vi "frequency_sweep_2.vi"() -> ()   [LabVIEW 2016]
uses:
  controls/State.ctl
  controls/Data.ctl
  <vilib>/Utility/error.llb/DialogType.ctl
  <vilib>/DAQmx/write.llb/DAQmx Write (Analog DBL 1Chan 1Samp).vi
  <vilib>/DAQmx/create/channels.llb/DAQmx Create Channel (AO-Voltage-Basic).vi
  <vilib>/DAQmx/miscellaneous.llb/DAQmx Fill In Error Info.vi
  <instrlib>/niVNA/niVNA.llb/niVNA Fetch Sweep Measurement (DBL).vi
panel:
  out "DAQ channel Out":tag="DAQ_6363/ao0"
  in  "Averaging Points":i32=4 min=1 max=3201 step=1
  in  "DAQ channel In":tag="DAQ_6363/ao0"
  in  "Exit Button":bool
  in  "IF Bandwidth":dbl(ring)=1000.0 items=["10 Hz"=10.0, "30 Hz"=30.0, "100 Hz"=100.0, "300 Hz"=300.0, "1 KHz"=1000.0, "3 KHz"=3000.0, "10 KHz"=10000.0, "30 KHz"=30000.0]
  in  "Reference H Field (Oe)":dbl=5500.0 min=-6000.0 max=6000.0
  in  "H Field (Oe)":dbl=1000.0 min=-6000.0 max=6000.0
  in  "Save Button":bool
  out "Status":string="Shutting down...Sweeping field to zero..."
  out "Cursor":cluster{"x":dbl, "y":dbl} {"x" format="%.2f"; "y" format="%.5f"}
  out "VNA Name Out":refnum<k15>="VNA_5630"
  out "Error Out":errorcluster
  in  "Error In (no error)":errorcluster
  in  "Format":i32(ring)=1 items=["Log Magnitude (dB)"=0, "Lin Magnitude"=1, "Phase (deg)"=2, "VSWR"=3, "Group Delay"=6]
  out "SpectrumGraph":cluster{"Field":dbl[], "Signal":dbl[]}(graph)
  in  "S-parameter":i32(ring)=1 caption="Measurement" items=["S11", "S21"]
  in  "Start Button":bool
  in  "Stop Button":bool
  in  "Output Power (dBm)":dbl=1.0 min=-25.0 max=5.0 step=0.5
  in  "Number of Points":i32=1000 min=1 max=3201 step=1
  in  "Stop frequency (GHz)":dbl=6.0 caption="Stop H Field (Oe)" min=0.01 max=6.0 format="%#_6f"
  in  "Start frequency (GHz)":dbl=1.0 min=0.01 max=6.0 format="%#_6f"
  in  "VNA Name In":refnum<k15>="VNA_5630"
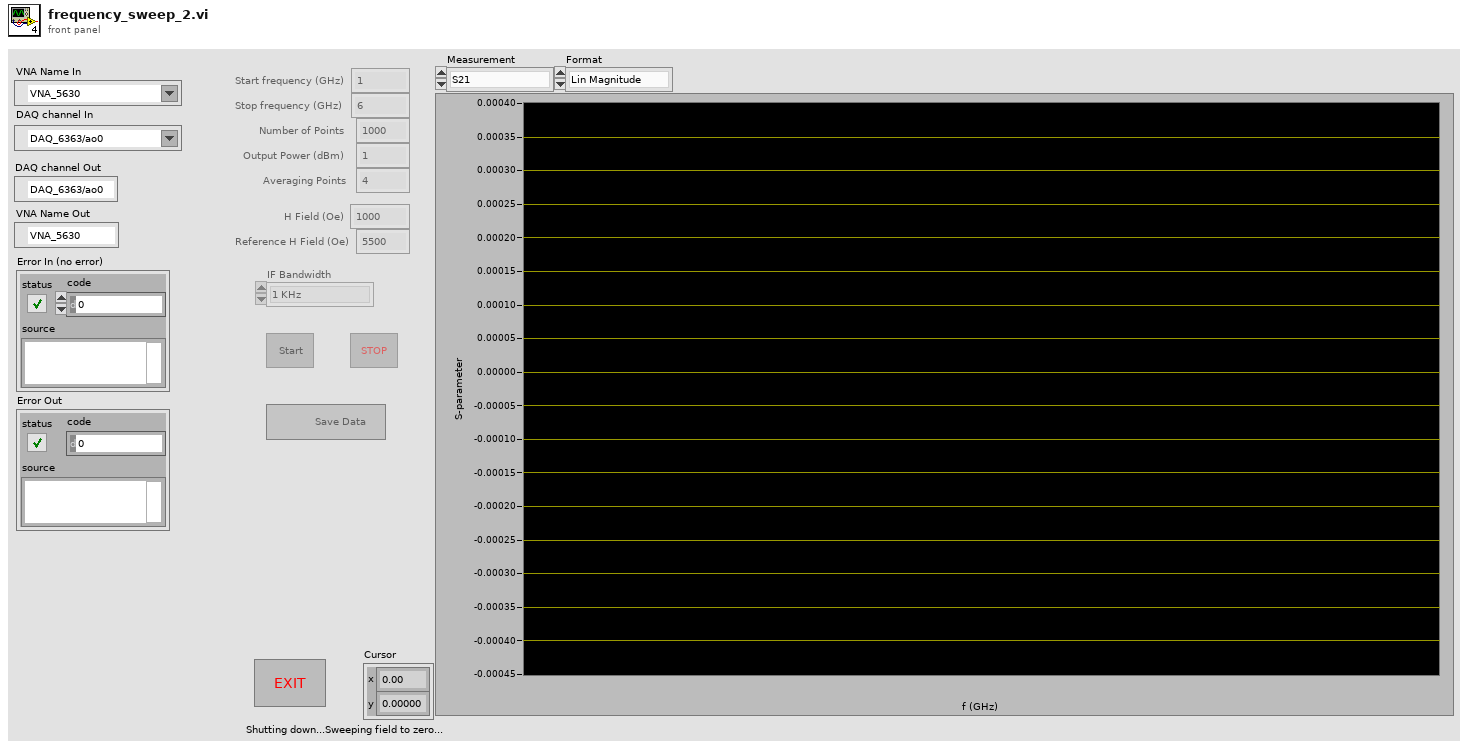
[diagram p1: front panel]
types:
  T1 = typedef "Data.ctl" = cluster{"Frequency":dbl[], "Signal":dbl[], "Ref signal":dbl[]}
  T2 = typedef "State.ctl" = enum16{"Init", "Idle", "Sweeping to ref", "Measuring ref", "Sweeping to H", "Measuring H", "Sweeping down", "Shutdown"}
  T3 = typedef "DialogType.ctl" = u16
  T4 = typedef "LVPoint32TypeDef.ctl" = cluster{"Horizontal":i32, "Vertical":i32}
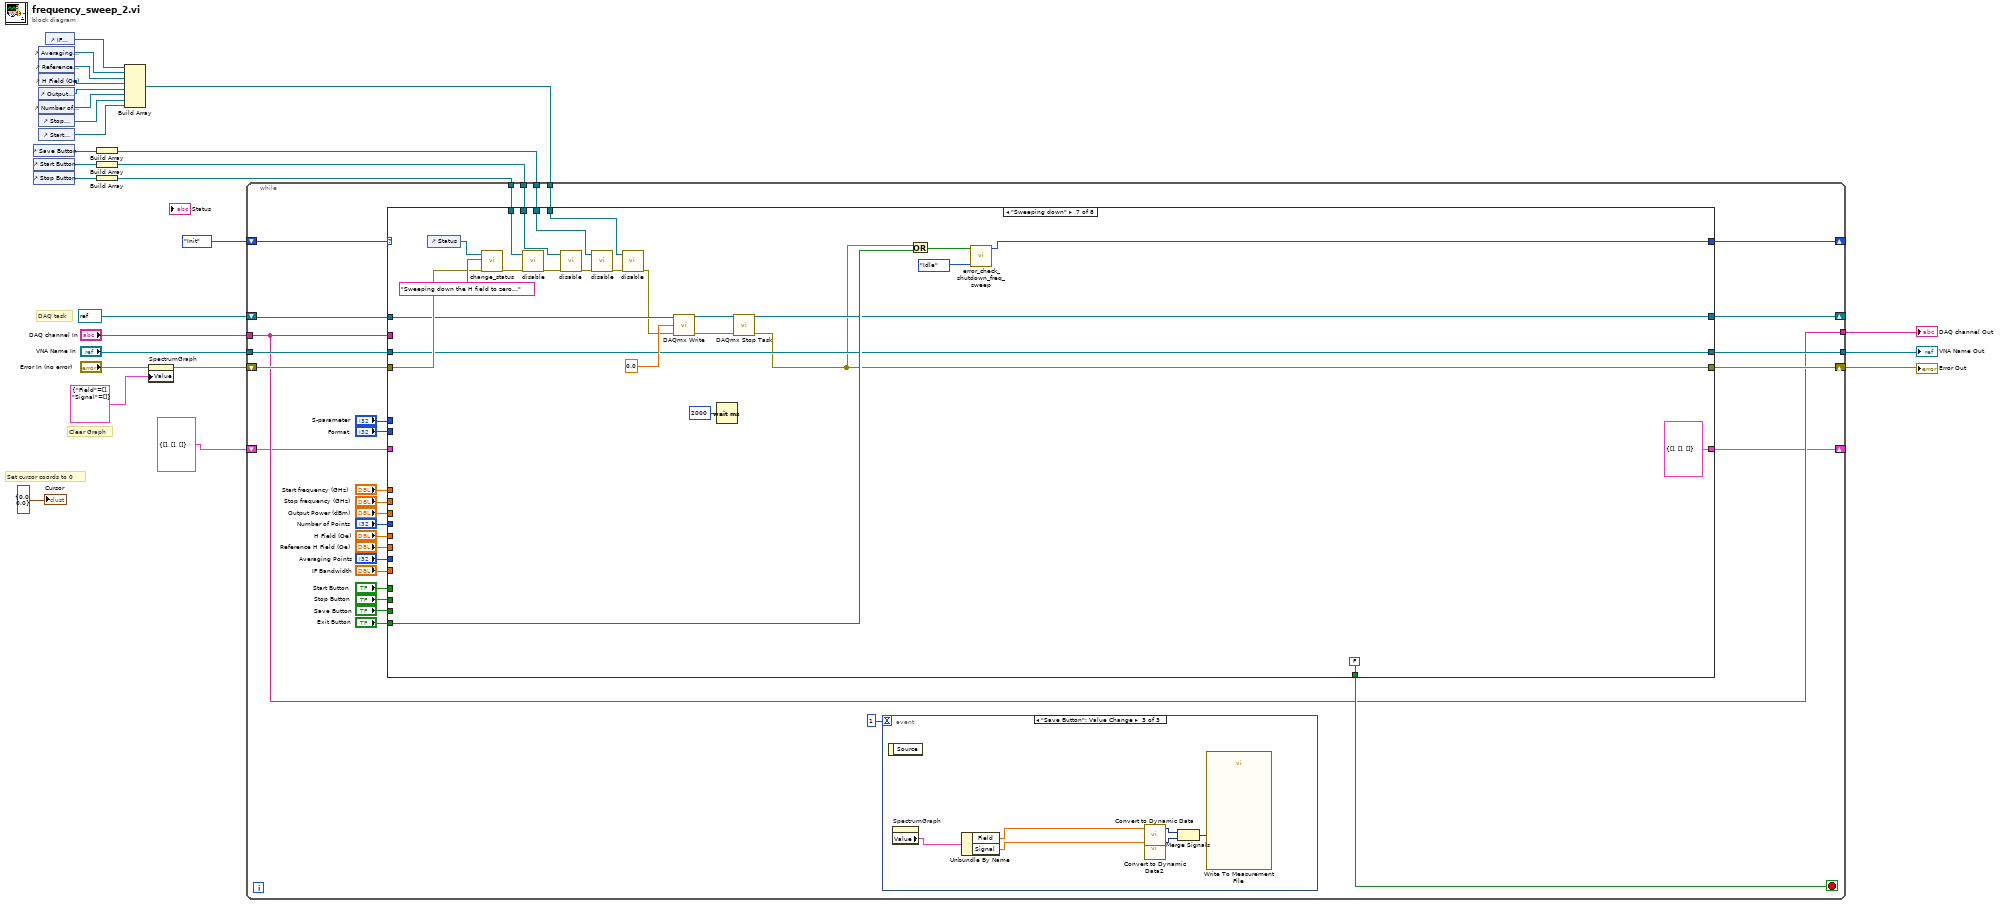
[diagram p0: block diagram]
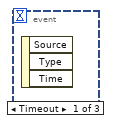
[diagram p2: hidden frame]
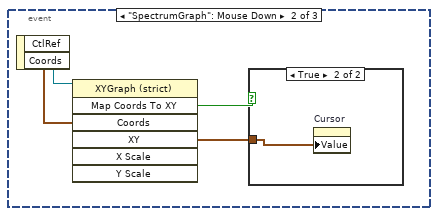
[diagram p3: hidden frame]
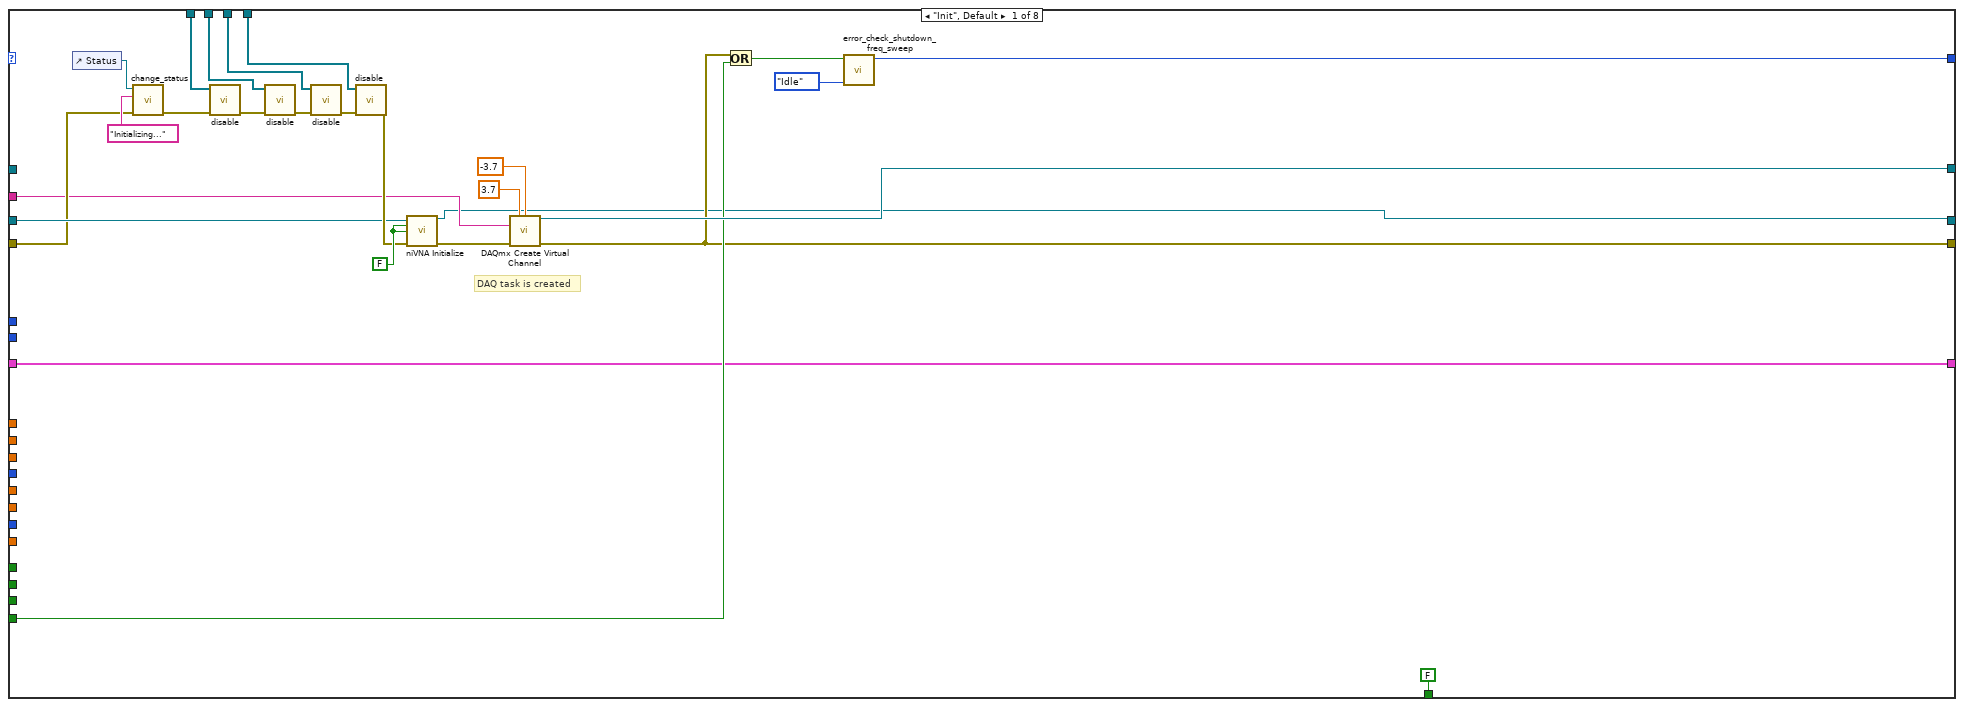
[diagram p5: hidden frame]
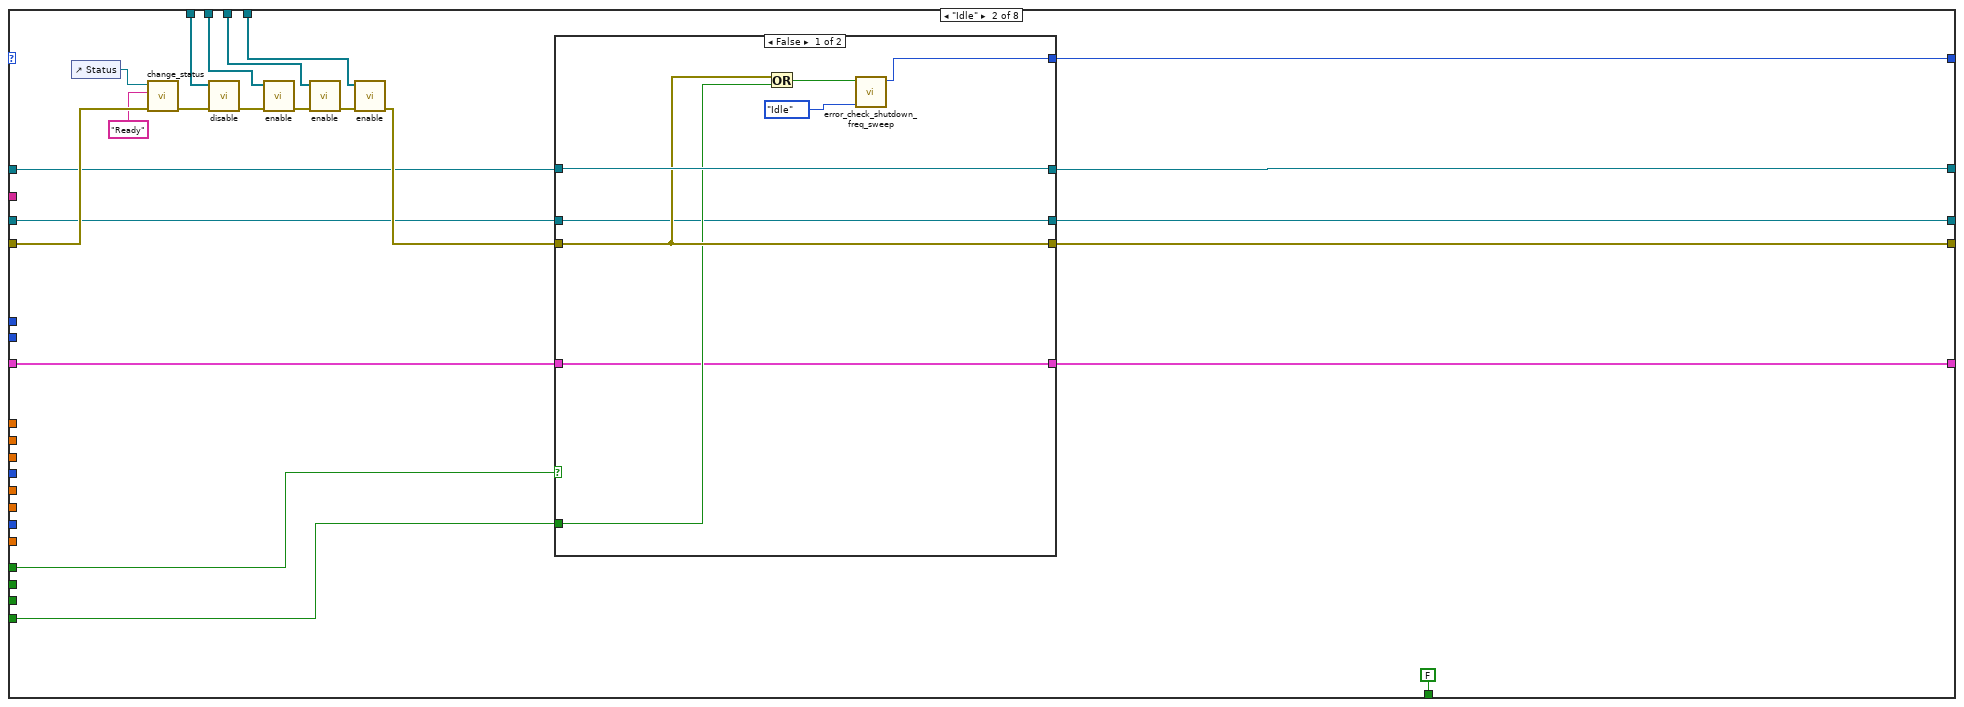
[diagram p6: hidden frame]
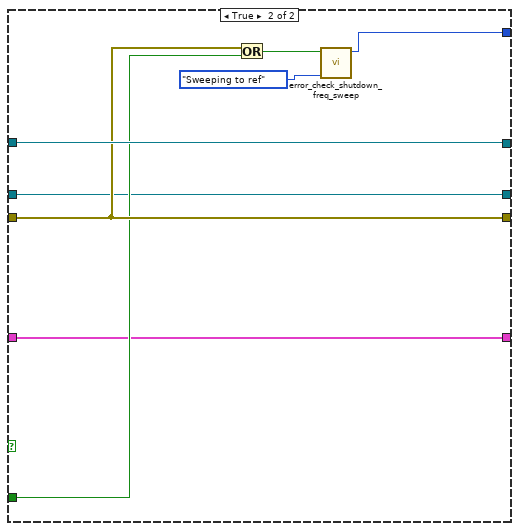
[diagram p7: hidden frame]
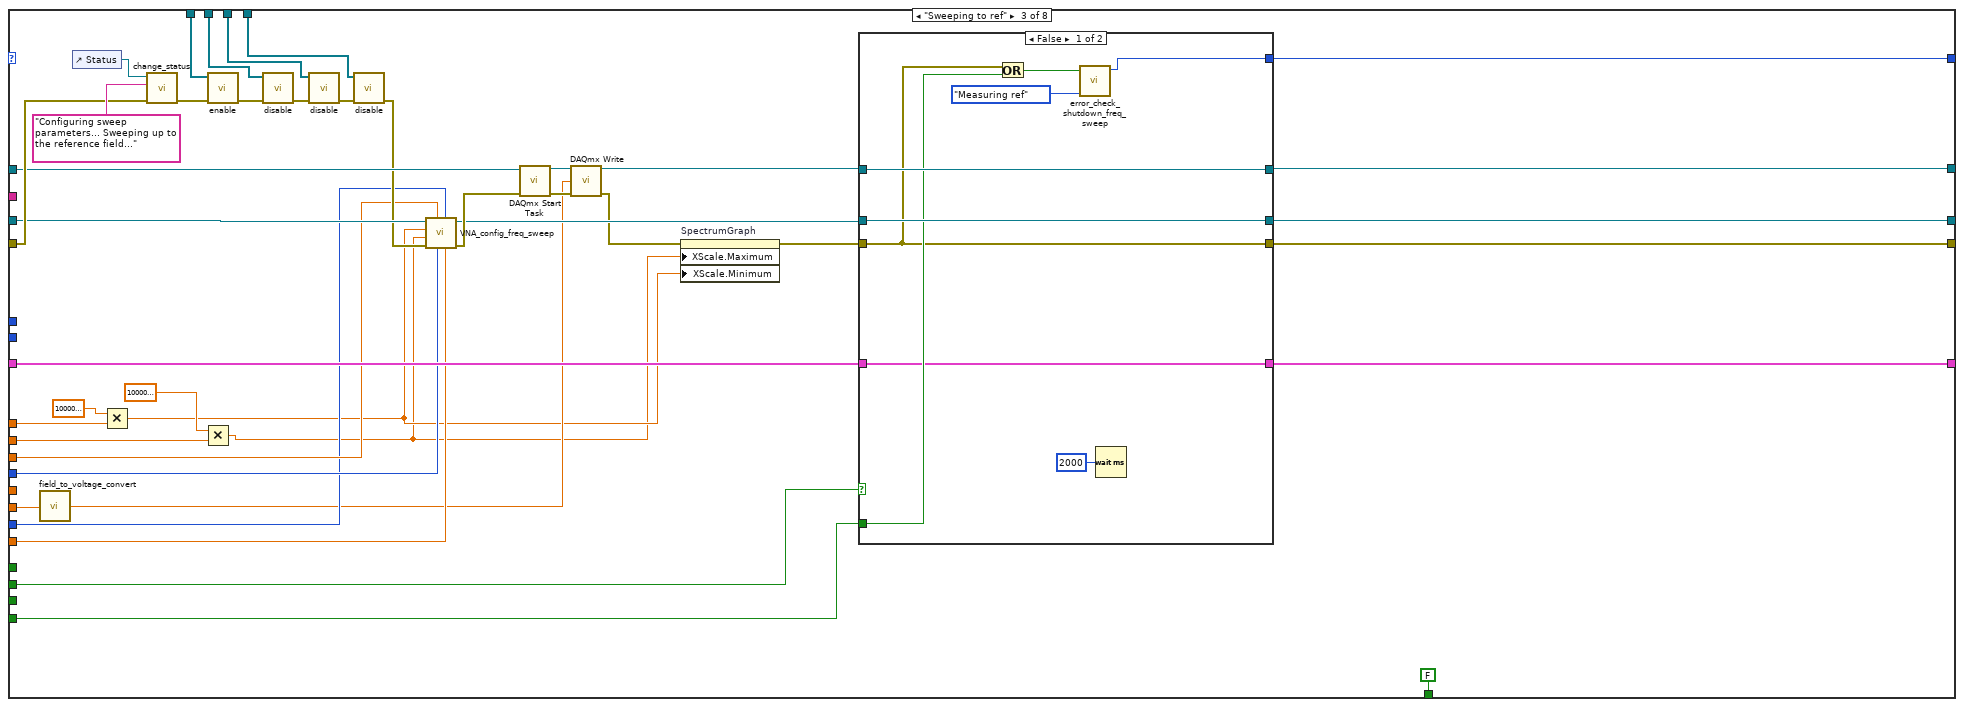
[diagram p8: hidden frame]
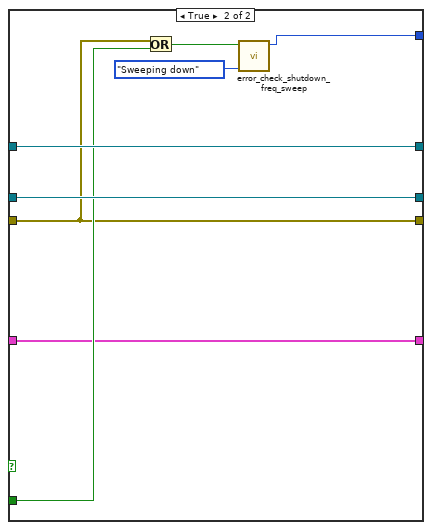
[diagram p9: hidden frame]
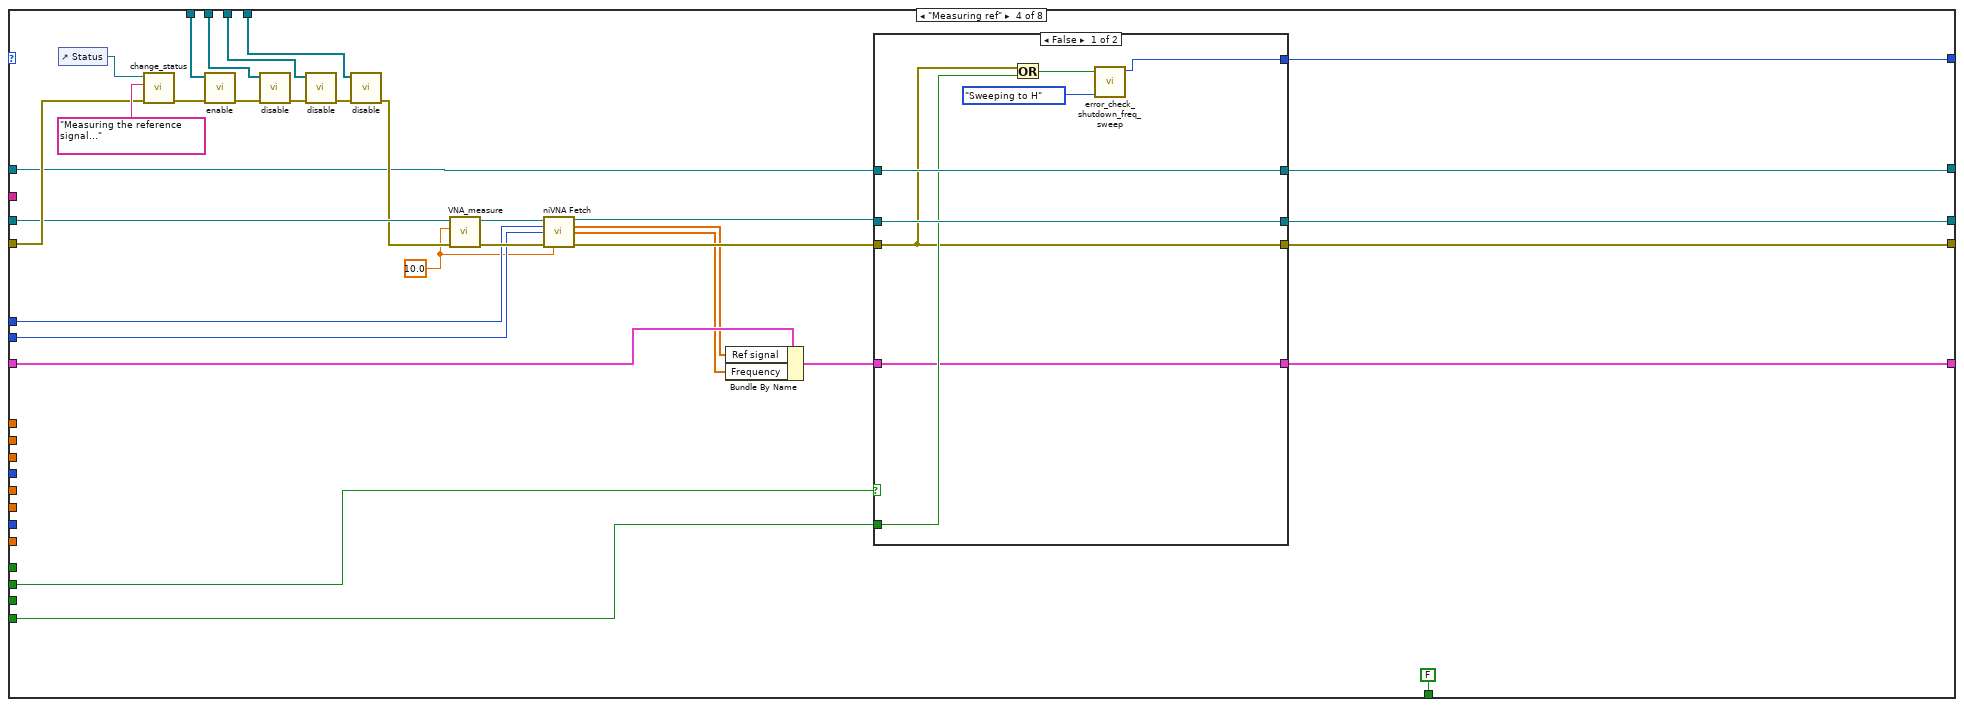
[diagram p10: hidden frame]
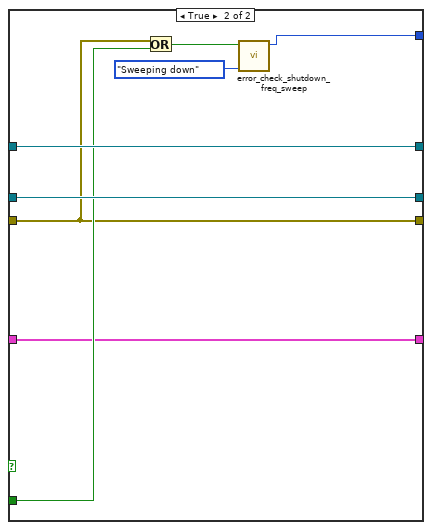
[diagram p11: hidden frame]
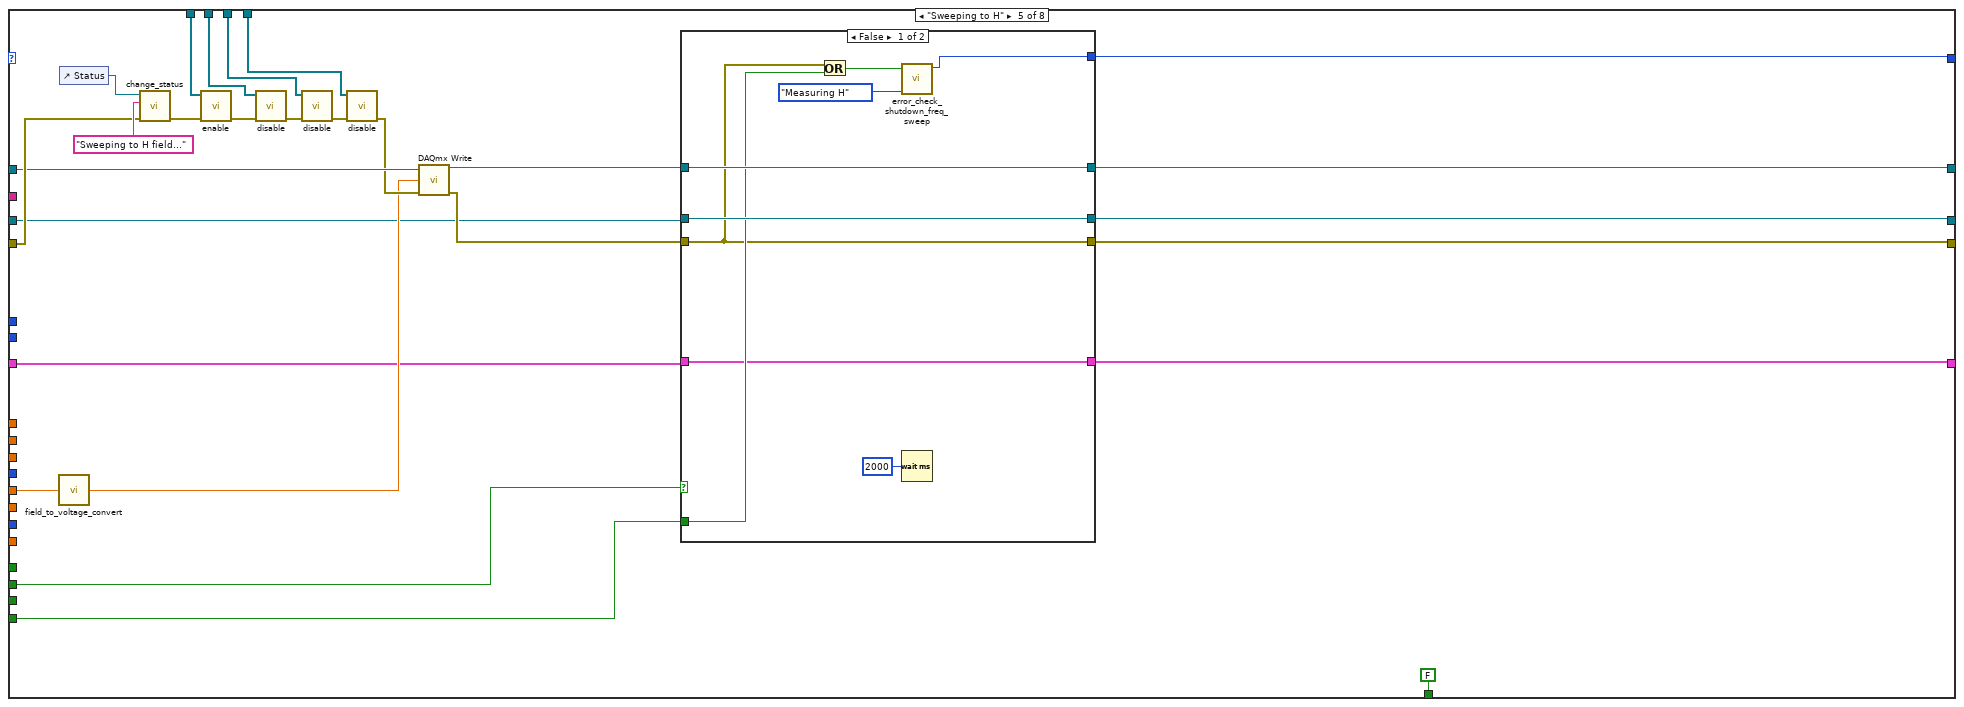
[diagram p12: hidden frame]
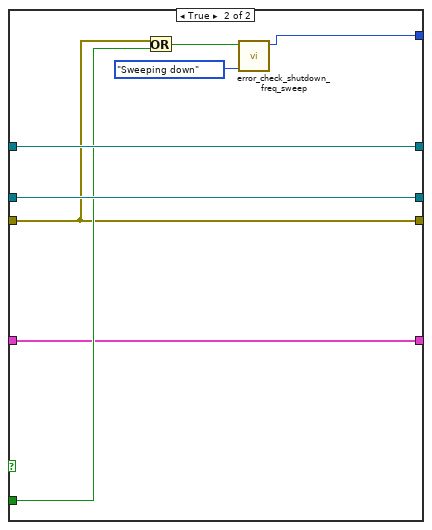
[diagram p13: hidden frame]
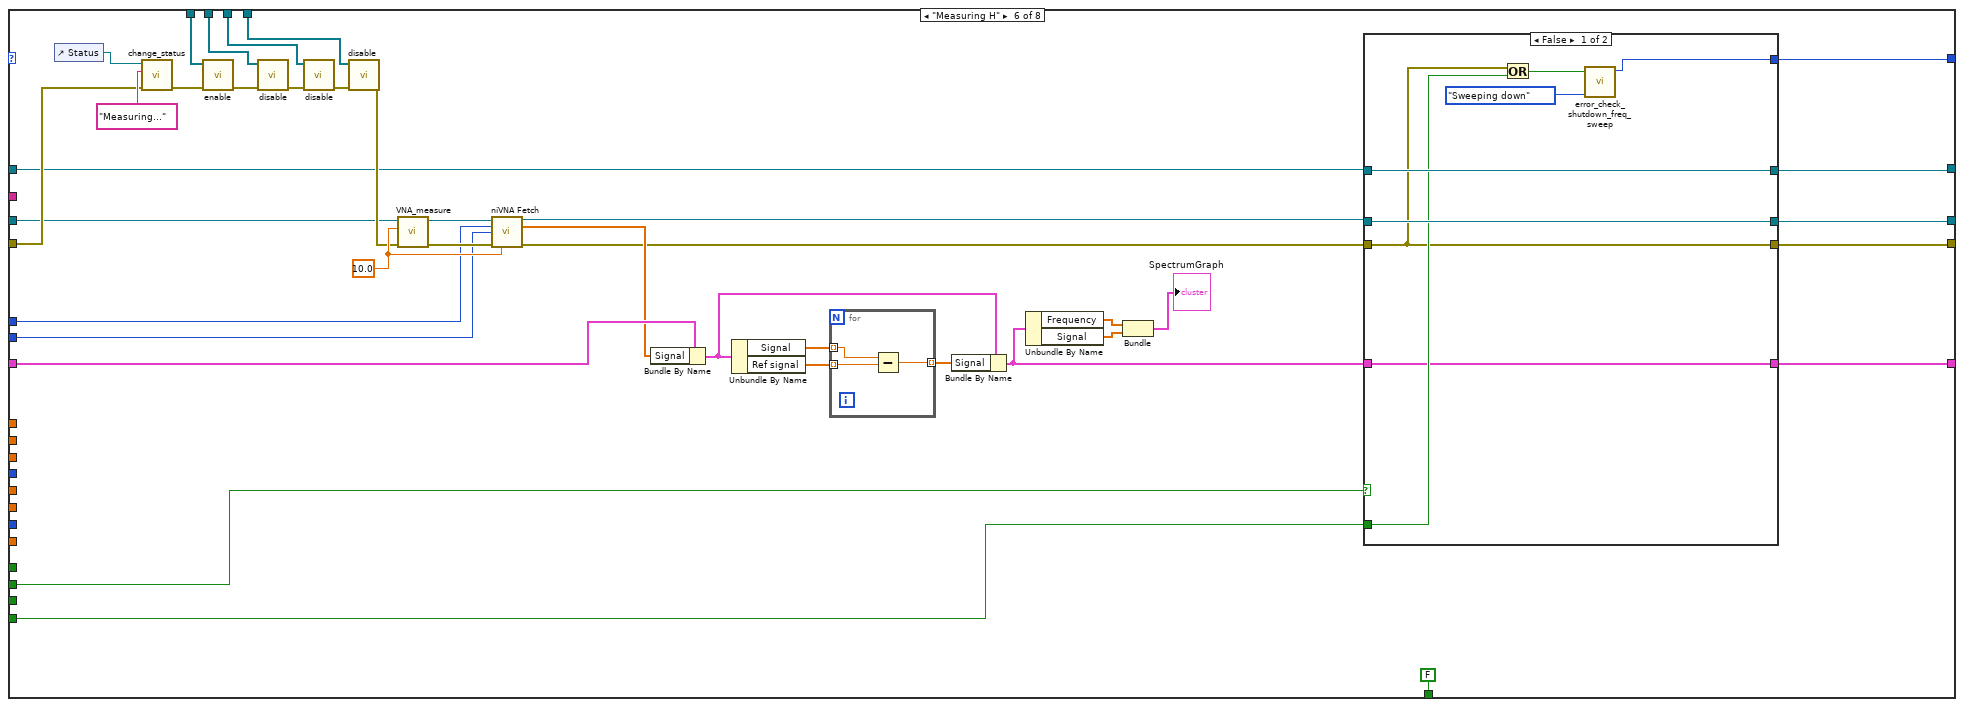
[diagram p14: hidden frame]
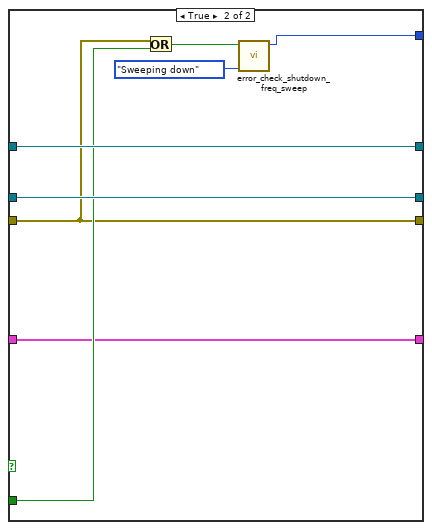
[diagram p15: hidden frame]
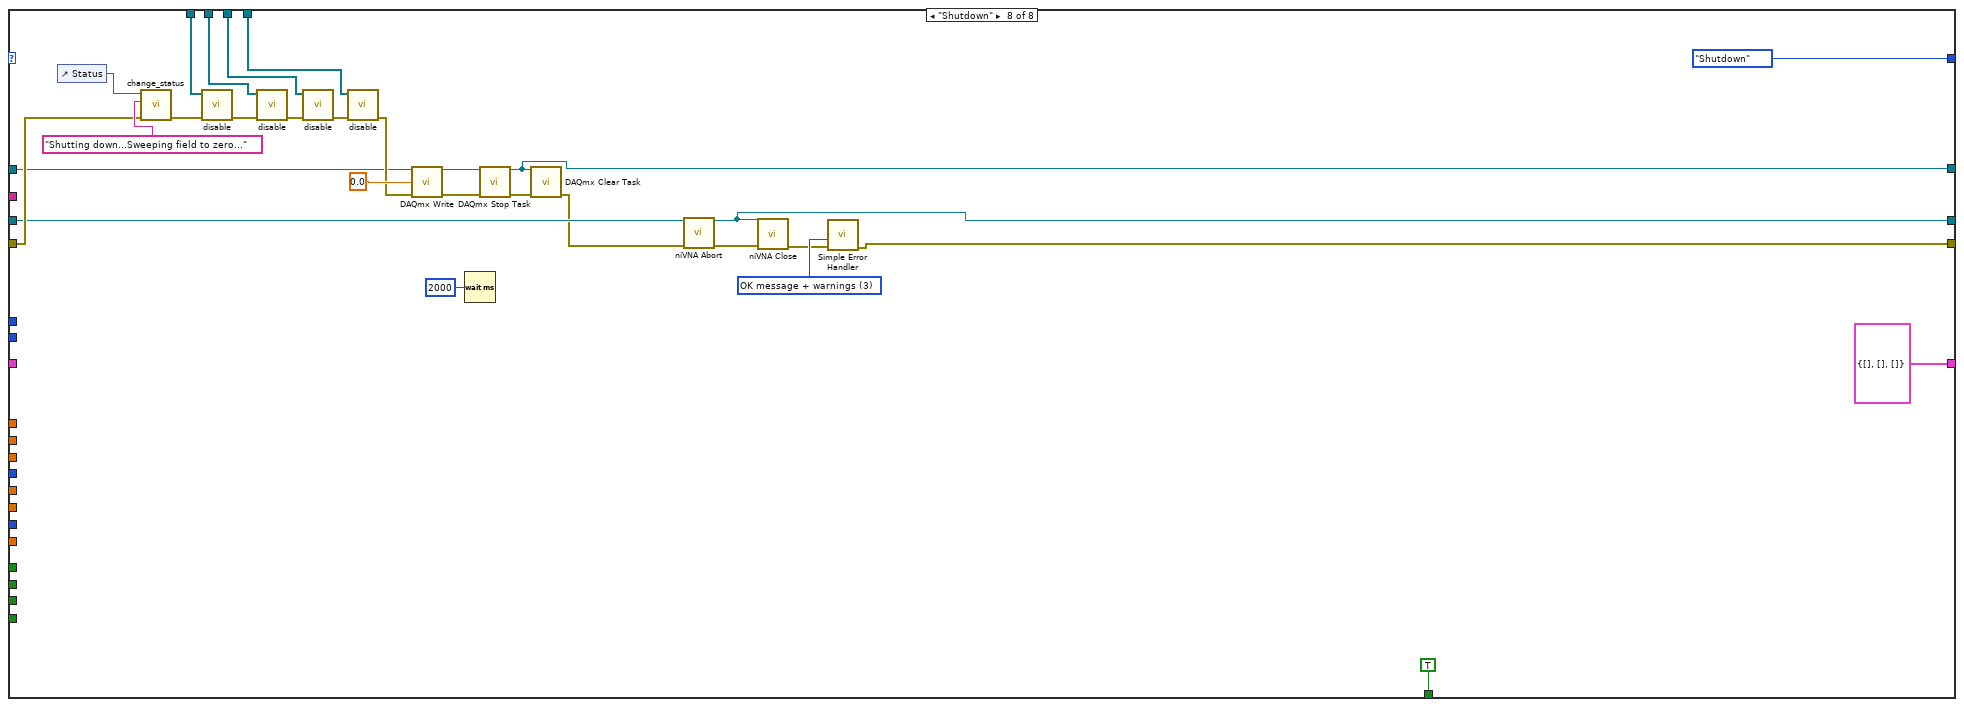
[diagram p16: hidden frame]
diagram:
  # "DAQ task"
  # "Set cursor coords to 0"
  # "Clear Graph"
  n1 = control-ref of="Save Button"() -> (w11:refnum<vi>)
  n2 = control-ref of="Start Button"() -> (w19:refnum<vi>)
  n3 = control-ref of="Stop Button"() -> (w18:refnum<vi>)
  n4 = control-ref of="Averaging Points"() -> (w9:refnum<vi>)
  n5 = control-ref of="Reference H Field (Oe)"() -> (w25:refnum<vi>)
  n6 = control-ref of="H Field (Oe)"() -> (w24:refnum<vi>)
  n7 = control-ref of="Output Power (dBm)"() -> (w23:refnum<vi>)
  n8 = control-ref of="Number of Points"() -> (w22:refnum<vi>)
  n9 = control-ref of="Stop frequency (GHz)"() -> (w21:refnum<vi>)
  n10 = control-ref of="Start frequency (GHz)"() -> (w20:refnum<vi>)
  n11 = control-ref of="IF Bandwidth"() -> (w26:refnum<vi>)
  n12 = Build Array(w11) -> (w10:refnum<vi>[])
  n13 = Build Array(w19) -> (w16:refnum<vi>[])
  n14 = Build Array(w18) -> (w15:refnum<vi>[])
  n15 = Build Array(w26, w9, w25, w24, w23, w22, w21, w20) -> (w17:refnum<vi>[])
  n16 = property on="SpectrumGraph" class="XYGraph (strict)"(error in="Error In (no error)", "Value"=cluster{"Field":dbl[], "Signal":dbl[]} {"Field"=[], "Signal"=[]} ("SpectrumGraph")) -> (error out=w4:errorcluster)  [unwired: 1 in, 1 out]
  n17 = while {
    shift-right: [w28] -> _
    shift-left: State."Init" -> [w31]
    tunnel: w17 -> [w58]
    tunnel: w16 -> [w57]
    tunnel: w15 -> [w56]
    tunnel: "VNA Name In" -> [w55]
    tunnel: "DAQ channel In" -> [w36]
    shift-right: [w54] -> w8
    shift-left: w4 -> [w53]
    shift-right: [w52] -> _
    shift-left: refnum<k21> refnum ("task in") -> [w51]
    tunnel: w10 -> [w50]
    tunnel: [w38] -> w7
    shift-right: [w32] -> _
    shift-left: T1 {"Frequency"=[], "Signal"=[], "Ref signal"=[]} -> [w33]
    tunnel: [w36] -> w6
    stop <- w45 stop-if-true
    n18 = case shown="\"Sweeping down\"" w31 {
      tunnel: w58 -> [w80 w116 w169 w224 w262 w318 w362 w391]
      tunnel: w57 -> [w94 w118 w171 w226 w264 w320 w360 w393]
      tunnel: w56 -> [w96 w119 w172 w227 w266 w321 w359 w394]
      tunnel: w55 -> [w88 w105 w156 w216 w252 w311 w355 w376]
      tunnel: w53 -> [w87 w111 w167 w217 w260 w317 w366 w389]
      tunnel: [w76 w97 w158 w204 w248 w289 w356 State."Shutdown" ("Enum")] -> w28
      tunnel: w36 -> [w83 _ _ _ _ _ _ _]
      tunnel: [w75 w106 w165 w201 w245 w292 w348 w384] -> w54
      tunnel: [w82 w103 w163 w203 w247 w290 w350 w385] -> w52
      tunnel: w51 -> [_ w104 w162 w206 w259 w295 w364 w379]
      tunnel: w50 -> [w81 w117 w170 w225 w263 w319 w361 w392]
      tunnel: "Start Button" -> [_ w108 _ _ _ _ _ _]
      tunnel: "Stop Button" -> [_ _ w166 w209 w250 w294 _ _]
      tunnel: "Save Button" -> [_ _ _ _ _ _ _ _]
      tunnel: "Exit Button" -> [w77 w102 w157 w208 w249 w293 w357 _]
      tunnel: [FALSE FALSE FALSE FALSE FALSE FALSE FALSE TRUE] -> w45
      tunnel: "Start frequency (GHz)" -> [_ _ w141 _ _ _ _ _]
      tunnel: "Stop frequency (GHz)" -> [_ _ w138 _ _ _ _ _]
      tunnel: "Output Power (dBm)" -> [_ _ w145 _ _ _ _ _]
      tunnel: "Number of Points" -> [_ _ w147 _ _ _ _ _]
      tunnel: "H Field (Oe)" -> [_ _ _ _ w256 _ _ _]
      tunnel: "Reference H Field (Oe)" -> [_ _ w143 _ _ _ _ _]
      tunnel: [w73 w101 w164 w202 w246 w291 w355 w386] -> w38
      tunnel: "Averaging Points" -> [_ _ w144 _ _ _ _ _]
      tunnel: w33 -> [w71 w100 w152 w199 w251 w308 _ _]
      tunnel: "IF Bandwidth" -> [_ _ w146 _ _ _ _ _]
      tunnel: [w71 w98 w148 w197 w244 w298 T1 {"Frequency"=[], "Signal"=[], "Ref signal"=[]} T1 {"Frequency"=[], "Signal"=[], "Ref signal"=[]}] -> w32
      tunnel: "S-parameter" -> [_ _ _ w212 _ w310 _ _]
      tunnel: "Format" -> [_ _ _ w211 _ w309 _ _]
      frame "Init", Default {
        w90 = FALSE ("id query")
        # "DAQ task is created"
        n19 = control-ref of="Status"() -> (w92:refnum<vi>)
        n20 = call "change_status.vi"("error in (no error)"=w87, "String"="Initializing...", "String in"=w92) -> ("error out"=w93:errorcluster)  [unwired: 8 in]
        n21 = call "disable.vi"("error in (no error)"=w93, "Array"=w96) -> ("error out"=w95:errorcluster)  [unwired: 9 in]
        n22 = call "disable.vi"("error in (no error)"=w95, "Array"=w94) -> ("error out"=w79:errorcluster)  [unwired: 9 in]
        n23 = call "disable.vi"("error in (no error)"=w79, "Array"=w81) -> ("error out"=w78:errorcluster)  [unwired: 9 in]
        n24 = call "disable.vi"("error in (no error)"=w78, "Array"=w80) -> ("error out"=w89:errorcluster)  [unwired: 9 in]
        n25 = call <instrlib>:"niVNA Initialize.vi"("resource name"=w88, "id query"=w90, "reset"=w90, "error in"=w89) -> ("instrument handle"=w73:refnum<k15>, "error out"=w86:errorcluster)  [unwired: 10 in]
        n26 = call-poly <vilib>:"DAQmx Create Virtual Channel.vi"("maximum value"=3.7, "minimum value"=-3.7, "physical channels"=w83, "error in"=w86) -> ("task out"=w82:refnum<k21>, "error out"=w75:errorcluster)  [unwired: 10 in]
        n27 = Or(x=w75, y=w77) -> (x .or. y?=w74:bool)
        n28 = call "error_check_shutdown_freq_sweep.vi"(8:State."Idle", "Boolean"=w74) -> (3:w76:T2)  [unwired: 9 in]
      }
      frame "Idle" {
        n29 = control-ref of="Status"() -> (w110:refnum<vi>)
        n30 = call "change_status.vi"("error in (no error)"=w111, "String"="Ready", "String in"=w110) -> ("error out"=w112:errorcluster)  [unwired: 8 in]
        n31 = call "disable.vi"("error in (no error)"=w112, "Array"=w119) -> ("error out"=w115:errorcluster)  [unwired: 9 in]
        n32 = call "enable.vi"("error in (no error)"=w115, "Array"=w118) -> ("error out"=w114:errorcluster)  [unwired: 9 in]
        n33 = call "enable.vi"("error in (no error)"=w114, "Array"=w117) -> ("error out"=w113:errorcluster)  [unwired: 9 in]
        n34 = call "enable.vi"("error in (no error)"=w113, "Array"=w116) -> ("error out"=w107:errorcluster)  [unwired: 9 in]
        n35 = case shown="False" w108 {
          tunnel: w107 -> [w126 w134]
          tunnel: [w126 w134] -> w106
          tunnel: w105 -> [w124 w132]
          tunnel: w104 -> [w127 w135]
          tunnel: [w127 w135] -> w103
          tunnel: [w120 w128] -> w97
          tunnel: w102 -> [w125 w133]
          tunnel: [w124 w132] -> w101
          tunnel: w100 -> [w123 w131]
          tunnel: [w123 w131] -> w98
          frame False {
            n36 = Or(x=w126, y=w125) -> (x .or. y?=w122:bool)
            n37 = call "error_check_shutdown_freq_sweep.vi"(8:State."Idle", "Boolean"=w122) -> (3:w120:T2)  [unwired: 9 in]
          }
          frame True {
            n38 = Or(x=w134, y=w133) -> (x .or. y?=w130:bool)
            n39 = call "error_check_shutdown_freq_sweep.vi"(8:State."Sweeping to ref", "Boolean"=w130) -> (3:w128:T2)  [unwired: 9 in]
          }
        }
      }
      frame "Sweeping to ref" {
        n40 = call "field_to_voltage_convert.vi"("Start H Field (Oe)"=w143) -> ("Numeric"=w142:dbl)
        n41 = control-ref of="Status"() -> (w168:refnum<vi>)
        n42 = Multiply(x=1000000000.0, y=w141) -> (x*y=w137:dbl)
        n43 = call "change_status.vi"("error in (no error)"=w167, "String"="Configuring sweep parameters... Sweeping up to the reference field...", "String in"=w168) -> ("error out"=w176:errorcluster)  [unwired: 8 in]
        n44 = Multiply(x=1000000000.0, y=w138) -> (x*y=w136:dbl)
        n45 = call "enable.vi"("error in (no error)"=w176, "Array"=w172) -> ("error out"=w175:errorcluster)  [unwired: 9 in]
        n46 = call "disable.vi"("error in (no error)"=w175, "Array"=w171) -> ("error out"=w174:errorcluster)  [unwired: 9 in]
        n47 = call "disable.vi"("error in (no error)"=w174, "Array"=w170) -> ("error out"=w173:errorcluster)  [unwired: 9 in]
        n48 = call "disable.vi"("error in (no error)"=w173, "Array"=w169) -> ("error out"=w155:errorcluster)  [unwired: 9 in]
        n49 = call "VNA_config_freq_sweep.vi"("IF Bandwidth"=w146, "Averaging"=w144, "Number of Points"=w147, "Output Power"=w145, "error in (no error)"=w155, "Stop Frequency"=w136, "Start Frequency"=w137, "Resource Name In"=w156) -> ("error out"=w154:errorcluster, "Resource Name Out"=w153:refnum<k15>)  [unwired: 2 in]
        n50 = call <vilib>:"DAQmx Start Task.vi"("task/channels in"=w162, "error in"=w154) -> ("task out"=w161:refnum<k21>, "error out"=w159:errorcluster)  [unwired: 12 in]
        n51 = call-poly <vilib>:"DAQmx Write.vi"("task/channels in"=w161, "data"=w142, "error in"=w159) -> ("task out"=w160:refnum<k21>, "error out"=w150:errorcluster)  [unwired: 10 in, 1 out]
        n52 = property on="SpectrumGraph" class="XYGraph (strict)"(error in=w150, "XScale.Maximum"=w136, "XScale.Minimum"=w137) -> (error out=w149:errorcluster)  [unwired: 1 in, 1 out]
        n53 = case shown="False" w166 {
          tunnel: w149 -> [w183 w191]
          tunnel: w160 -> [w186 w193]
          tunnel: w153 -> [w185 w194]
          tunnel: [w183 w191] -> w165
          tunnel: [w185 w194] -> w164
          tunnel: [w186 w193] -> w163
          tunnel: [w178 w188] -> w158
          tunnel: w157 -> [w184 w192]
          tunnel: w152 -> [w181 w190]
          tunnel: [w181 w190] -> w148
          frame False {
            n54 = Or(x=w183, y=w184) -> (x .or. y?=w180:bool)
            n55 = call "error_check_shutdown_freq_sweep.vi"(8:State."Measuring ref", "Boolean"=w180) -> (3:w178:T2)  [unwired: 9 in]
            n56 = Wait (ms)(milliseconds to wait=u32 2000) -> ()  [unwired: 1 out]
          }
          frame True {
            n57 = Or(x=w191, y=w192) -> (x .or. y?=w189:bool)
            n58 = call "error_check_shutdown_freq_sweep.vi"(8:State."Sweeping down", "Boolean"=w189) -> (3:w188:T2)  [unwired: 9 in]
          }
        }
      }
      frame "Measuring ref" {
        w210 = 10.0 ("timeout")
        n59 = control-ref of="Status"() -> (w218:refnum<vi>)
        n60 = call "change_status.vi"("error in (no error)"=w217, "String"="Measuring the reference signal...", "String in"=w218) -> ("error out"=w223:errorcluster)  [unwired: 8 in]
        n61 = call "enable.vi"("error in (no error)"=w223, "Array"=w227) -> ("error out"=w222:errorcluster)  [unwired: 9 in]
        n62 = call "disable.vi"("error in (no error)"=w222, "Array"=w226) -> ("error out"=w221:errorcluster)  [unwired: 9 in]
        n63 = call "disable.vi"("error in (no error)"=w221, "Array"=w225) -> ("error out"=w220:errorcluster)  [unwired: 9 in]
        n64 = call "disable.vi"("error in (no error)"=w220, "Array"=w224) -> ("error out"=w215:errorcluster)  [unwired: 9 in]
        n65 = call "VNA_measure.vi"("error in (no error)"=w215, "timeout"=w210, "Resource Name In"=w216) -> ("error out"=w213:errorcluster, "Resource Name Out"=w214:refnum<k15>)  [unwired: 7 in]
        n66 = call-poly <instrlib>:"niVNA Fetch.vi"("instrument handle"=w214, "measurement"=w212, "format"=w211, "error in"=w213, "timeout"=w210) -> ("instrument handle out"=w205:refnum<k15>, "data"=w196:dbl[], "scale points"=w195:dbl[], "error out"=w207:errorcluster)  [unwired: 7 in]
        n67 = Bundle By Name(cluster=w199, "Ref signal"=w196, "Frequency"=w195) -> (w198:T1)
        n68 = case shown="False" w209 {
          tunnel: w207 -> [w232 w240]
          tunnel: w206 -> [w235 w242]
          tunnel: w205 -> [w234 w243]
          tunnel: [w232 w240] -> w201
          tunnel: [w234 w243] -> w202
          tunnel: [w235 w242] -> w203
          tunnel: [w229 w238] -> w204
          tunnel: w208 -> [w233 w241]
          tunnel: [w228 w236] -> w197
          tunnel: w198 -> [w228 w236]
          frame False {
            n69 = Or(x=w232, y=w233) -> (x .or. y?=w231:bool)
            n70 = call "error_check_shutdown_freq_sweep.vi"(8:State."Sweeping to H", "Boolean"=w231) -> (3:w229:T2)  [unwired: 9 in]
          }
          frame True {
            n71 = Or(x=w240, y=w241) -> (x .or. y?=w239:bool)
            n72 = call "error_check_shutdown_freq_sweep.vi"(8:State."Sweeping down", "Boolean"=w239) -> (3:w238:T2)  [unwired: 9 in]
          }
        }
      }
      frame "Sweeping to H" {
        n73 = call "field_to_voltage_convert.vi"("Start H Field (Oe)"=w256) -> ("Numeric"=w255:dbl)
        n74 = control-ref of="Status"() -> (w261:refnum<vi>)
        n75 = call "change_status.vi"("error in (no error)"=w260, "String"="Sweeping to H field...", "String in"=w261) -> ("error out"=w267:errorcluster)  [unwired: 8 in]
        n76 = call "enable.vi"("error in (no error)"=w267, "Array"=w266) -> ("error out"=w270:errorcluster)  [unwired: 9 in]
        n77 = call "disable.vi"("error in (no error)"=w270, "Array"=w264) -> ("error out"=w269:errorcluster)  [unwired: 9 in]
        n78 = call "disable.vi"("error in (no error)"=w269, "Array"=w263) -> ("error out"=w268:errorcluster)  [unwired: 9 in]
        n79 = call "disable.vi"("error in (no error)"=w268, "Array"=w262) -> ("error out"=w258:errorcluster)  [unwired: 9 in]
        n80 = call-poly <vilib>:"DAQmx Write.vi"("task/channels in"=w259, "data"=w255, "error in"=w258) -> ("task out"=w253:refnum<k21>, "error out"=w254:errorcluster)  [unwired: 10 in, 1 out]
        n81 = case shown="False" w250 {
          tunnel: w254 -> [w276 w284]
          tunnel: w253 -> [w279 w286]
          tunnel: w252 -> [w278 w287]
          tunnel: [w276 w284] -> w245
          tunnel: [w278 w287] -> w246
          tunnel: [w279 w286] -> w247
          tunnel: [w272 w281] -> w248
          tunnel: w249 -> [w277 w285]
          tunnel: w251 -> [w275 w283]
          tunnel: [w275 w283] -> w244
          frame False {
            n82 = Or(x=w276, y=w277) -> (x .or. y?=w274:bool)
            n83 = call "error_check_shutdown_freq_sweep.vi"(8:State."Measuring H", "Boolean"=w274) -> (3:w272:T2)  [unwired: 9 in]
            n84 = Wait (ms)(milliseconds to wait=u32 2000) -> ()  [unwired: 1 out]
          }
          frame True {
            n85 = Or(x=w284, y=w285) -> (x .or. y?=w282:bool)
            n86 = call "error_check_shutdown_freq_sweep.vi"(8:State."Sweeping down", "Boolean"=w282) -> (3:w281:T2)  [unwired: 9 in]
          }
        }
      }
      frame "Measuring H" {
        w313 = 10.0 ("timeout")
        n87 = control-ref of="Status"() -> (w316:refnum<vi>)
        n88 = call "change_status.vi"("error in (no error)"=w317, "String"="Measuring...", "String in"=w316) -> ("error out"=w326:errorcluster)  [unwired: 8 in]
        n89 = call "enable.vi"("error in (no error)"=w326, "Array"=w321) -> ("error out"=w325:errorcluster)  [unwired: 9 in]
        n90 = call "disable.vi"("error in (no error)"=w325, "Array"=w320) -> ("error out"=w324:errorcluster)  [unwired: 9 in]
        n91 = call "disable.vi"("error in (no error)"=w324, "Array"=w319) -> ("error out"=w323:errorcluster)  [unwired: 9 in]
        n92 = call "disable.vi"("error in (no error)"=w323, "Array"=w318) -> ("error out"=w312:errorcluster)  [unwired: 9 in]
        n93 = call "VNA_measure.vi"("error in (no error)"=w312, "timeout"=w313, "Resource Name In"=w311) -> ("error out"=w314:errorcluster, "Resource Name Out"=w315:refnum<k15>)  [unwired: 7 in]
        n94 = call-poly <instrlib>:"niVNA Fetch.vi"("instrument handle"=w315, "measurement"=w310, "format"=w309, "error in"=w314, "timeout"=w313) -> ("instrument handle out"=w296:refnum<k15>, "data"=w307:dbl[], "error out"=w297:errorcluster)  [unwired: 7 in, 1 out]
        n95 = Bundle By Name(cluster=w308, "Signal"=w307) -> (w304:T1)
        n96 = Unbundle By Name(w304) -> ("Signal"=w306:dbl[], "Ref signal"=w305:dbl[])
        n97 = for {
          tunnel: w306 -> [w345] mode=indexing
          tunnel: w305 -> [w344] mode=indexing
          tunnel: [w343] -> w303 mode=indexing
          n98 = Subtract(x=w345, y=w344) -> (x-y=w343:dbl)
        }
        n99 = Bundle By Name(cluster=w304, "Signal"=w303) -> (w299:T1)
        n100 = Unbundle By Name(w299) -> ("Frequency"=w302:dbl[], "Signal"=w301:dbl[])
        n101 = Bundle("Frequency"=w302, "Signal"=w301) -> (→"SpectrumGraph":cluster{"Frequency":dbl[], "Signal":dbl[]})  [unwired: 1 in]
        n102 = case shown="False" w294 {
          tunnel: w297 -> [w331 w339]
          tunnel: w295 -> [w334 w341]
          tunnel: w296 -> [w333 w342]
          tunnel: [w331 w339] -> w292
          tunnel: [w333 w342] -> w291
          tunnel: [w334 w341] -> w290
          tunnel: [w328 w337] -> w289
          tunnel: w293 -> [w332 w340]
          tunnel: [w327 w335] -> w298
          tunnel: w299 -> [w327 w335]
          frame False {
            n103 = Or(x=w331, y=w332) -> (x .or. y?=w330:bool)
            n104 = call "error_check_shutdown_freq_sweep.vi"(8:State."Sweeping down", "Boolean"=w330) -> (3:w328:T2)  [unwired: 9 in]
          }
          frame True {
            n105 = Or(x=w339, y=w340) -> (x .or. y?=w338:bool)
            n106 = call "error_check_shutdown_freq_sweep.vi"(8:State."Sweeping down", "Boolean"=w338) -> (3:w337:T2)  [unwired: 9 in]
          }
        }
      }
      frame "Sweeping down" {
        n107 = control-ref of="Status"() -> (w354:refnum<vi>)
        n108 = call "change_status.vi"("error in (no error)"=w366, "String"="Sweeping down the H field to zero...", "String in"=w354) -> ("error out"=w370:errorcluster)  [unwired: 8 in]
        n109 = call "disable.vi"("error in (no error)"=w370, "Array"=w359) -> ("error out"=w369:errorcluster)  [unwired: 9 in]
        n110 = call "disable.vi"("error in (no error)"=w369, "Array"=w360) -> ("error out"=w368:errorcluster)  [unwired: 9 in]
        n111 = call "disable.vi"("error in (no error)"=w368, "Array"=w361) -> ("error out"=w367:errorcluster)  [unwired: 9 in]
        n112 = call "disable.vi"("error in (no error)"=w367, "Array"=w362) -> ("error out"=w363:errorcluster)  [unwired: 9 in]
        n113 = call-poly <vilib>:"DAQmx Write.vi"("task/channels in"=w364, "data"=0.0, "error in"=w363) -> ("task out"=w351:refnum<k21>, "error out"=w349:errorcluster)  [unwired: 10 in, 1 out]
        n114 = Wait (ms)(milliseconds to wait=u32 2000) -> ()  [unwired: 1 out]
        n115 = call <vilib>:"DAQmx Stop Task.vi"("task/channels in"=w351, "error in"=w349) -> ("task out"=w350:refnum<k21>, "error out"=w348:errorcluster)  [unwired: 12 in]
        n116 = Or(x=w348, y=w357) -> (x .or. y?=w358:bool)
        n117 = call "error_check_shutdown_freq_sweep.vi"(8:State."Idle", "Boolean"=w358) -> (3:w356:T2)  [unwired: 9 in]
      }
      frame "Shutdown" {
        w383 = T3 3 items=["no dialog", "OK message", "continue or stop message", "OK message + warnings", "continue/stop + warnings"] ("type of dialog (OK msg:1)")
        n118 = control-ref of="Status"() -> (w390:refnum<vi>)
        n119 = call "change_status.vi"("error in (no error)"=w389, "String"="Shutting down...Sweeping field to zero...", "String in"=w390) -> ("error out"=w396:errorcluster)  [unwired: 8 in]
        n120 = call "disable.vi"("error in (no error)"=w396, "Array"=w394) -> ("error out"=w399:errorcluster)  [unwired: 9 in]
        n121 = call "disable.vi"("error in (no error)"=w399, "Array"=w393) -> ("error out"=w398:errorcluster)  [unwired: 9 in]
        n122 = call "disable.vi"("error in (no error)"=w398, "Array"=w392) -> ("error out"=w397:errorcluster)  [unwired: 9 in]
        n123 = call "disable.vi"("error in (no error)"=w397, "Array"=w391) -> ("error out"=w380:errorcluster)  [unwired: 9 in]
        n124 = call-poly <vilib>:"DAQmx Write.vi"("task/channels in"=w379, "data"=0.0, "error in"=w380) -> ("task out"=w377:refnum<k21>, "error out"=w378:errorcluster)  [unwired: 10 in, 1 out]
        n125 = Wait (ms)(milliseconds to wait=u32 2000) -> ()  [unwired: 1 out]
        n126 = call <vilib>:"DAQmx Stop Task.vi"("task/channels in"=w377, "error in"=w378) -> ("task out"=w385:refnum<k21>, "error out"=w387:errorcluster)  [unwired: 12 in]
        n127 = call <vilib>:"DAQmx Clear Task.vi"("task in"=w385, "error in"=w387) -> ("error out"=w375:errorcluster)  [unwired: 13 in]
        n128 = call <instrlib>:"niVNA Abort.vi"("instrument handle"=w376, "error in"=w375) -> ("instrument handle out"=w386:refnum<k15>, "error out"=w388:errorcluster)  [unwired: 12 in]
        n129 = call <instrlib>:"niVNA Close.vi"("instrument handle"=w386, "error in"=w388) -> ("error out"=w374:errorcluster)  [unwired: 13 in]
        n130 = call <vilib>:"Simple Error Handler.vi"("type of dialog (OK msg:1)"=w383, "error in (no error)"=w374) -> ("error out"=w384:errorcluster)  [unwired: 3 in, 4 out]
      }
    }
    n131 = event shown="[2] \"Save Button\": Value Change" {
      selector: _ -> [_ _ _]
      dyn-events: _ -> [_ _ _]
      timeout: 1 -> [_ _ _]
      event Timeout {
        n132 = event-data() -> ()  [unwired: 1 in, 3 out]
      }
      event "SpectrumGraph": Mouse Down {
        n133 = event-data() -> ("CtlRef"=w59:refnum<vi>, "Coords"=w60:T4)  [unwired: 1 in]
        n134 = invoke on="Invoke Node" class="XYGraph (strict)" method="Map Coords To XY"(reference=w59, "Coords"=w60) -> ("Map Coords To XY"=w61:bool, "XY"=w62:cluster{"X":dbl, "Y":dbl})  [unwired: 5 in, 5 out]
        n135 = case shown="True" w61 {
          tunnel: w62 -> [_ w63]
          frame False {
          }
          frame True {
            n136 = property on="Cursor" class="Clust (strict)"("Value"=w63) -> ()  [unwired: 2 in, 2 out]
          }
        }
      }
      event "Save Button": Value Change {
        n137 = event-data() -> ()  [unwired: 1 in, 1 out]
        n138 = property on="SpectrumGraph" class="XYGraph (strict)"() -> ("Value"=w64:cluster{"Field":dbl[], "Signal":dbl[]})  [unwired: 2 in, 2 out]
        n139 = Unbundle By Name(w64) -> ("Field"=w66:dbl[], "Signal"=w65:dbl[])
        n140 = call "Convert to Dynamic Data"("Array"=w66) -> ("Dynamic Data Type"=w69:dynamicdata)  [unwired: 3 in]
        n141 = call "Convert to Dynamic Data2"("Array"=w65) -> ("Dynamic Data Type"=w67:dynamicdata)  [unwired: 3 in]
        n142 = Merge Signals(w69, w67) -> (w68:dynamicdata)
        n143 = call "Write To Measurement File"("Signals"=w68) -> ()  [unwired: 16 in, 3 out]
      }
    }
  }
  "Error Out" <- w8
  "VNA Name Out" <- w7
  "DAQ channel Out" <- w6
  "Cursor" <- cluster{"x":dbl, "y":dbl} {"x"=0.0, "y"=0.0} ("Cursor")
